vi "Local MS Initialization.vi"(6 "PID Cluster":T2={"L1 to L4 PID Cluster"={"L1 PID Gains"={"Kp"=0.005, "Kd"=0.5, "Ki"=0.0005}, "L2 PID Gains"={"Kp"=0.01, "Kd"=1.0, "Ki"=0.005}, "L3 PID Gains"={"Kp"=0.05, "Kd"=1.0, "Ki"=0.0005}, "L4 PID Gains"={"Kp"=0.1, "Kd"=0.1, "Ki"=0.0005}}, "Stage PID Cluster"={"Stage Z PID"={"Kp"=0.0005, "Kd"=0.001, "Ki"=0.0}, "Stage Y PID"={"Kp"=0.0003, "Kd"=0.01, "Ki"=0.0}, "Stage X PID"={"Kp"=0.0003, "Kd"=0.01, "Ki"=0.0}}, "OCT Z PID Gains"={"Kp"=0.0003, "Kd"=0.0001, "Ki"=0.01}}, 8 "error in":errorcluster, 9 "Offset Home 2 RCM":dbl[](array[numeric])=[0.0, 0.0, 0.0, 0.0], 10 "Prev Posit Cluster":T3={"Prev L1 to L4 Posit"=[0.0, 0.0, 0.0, 0.0], "Prev Stage Posit"=[6.0, 6.0, 6.0], "Prev OCT Z Posit"=0.0}, 11 "FPGA VI Reference In":refnum<k20>) -> (0 "error out":errorcluster, 2 "Last Posit Cluster":T1={"Last L1 to L4 Posit"=[0.0, 0.0, 0.0, 0.0], "Last Stage Posit"=[6.0, 6.0, 6.0], "Last OCT Z Posit"=0.0}, 3 "FPGA VI Reference Out":refnum<k20>)   [LabVIEW 2016]
uses:
  <vilib>/Platform/TimedLoop/XDataNode/timing_clust.ctl
  <vilib>/Platform/TimedLoop/XDataNode/nitl_modes.ctl
  <vilib>/Platform/TimedLoop/XDataNode/wakeup.ctl
  Global Variables.vi
  <vilib>/platform/TimedLoop/XDataNode/XDataNode.xnode
  <vilib>/Platform/TimedLoop/XDataNode/XDNodeRunTimeDep.lvlib
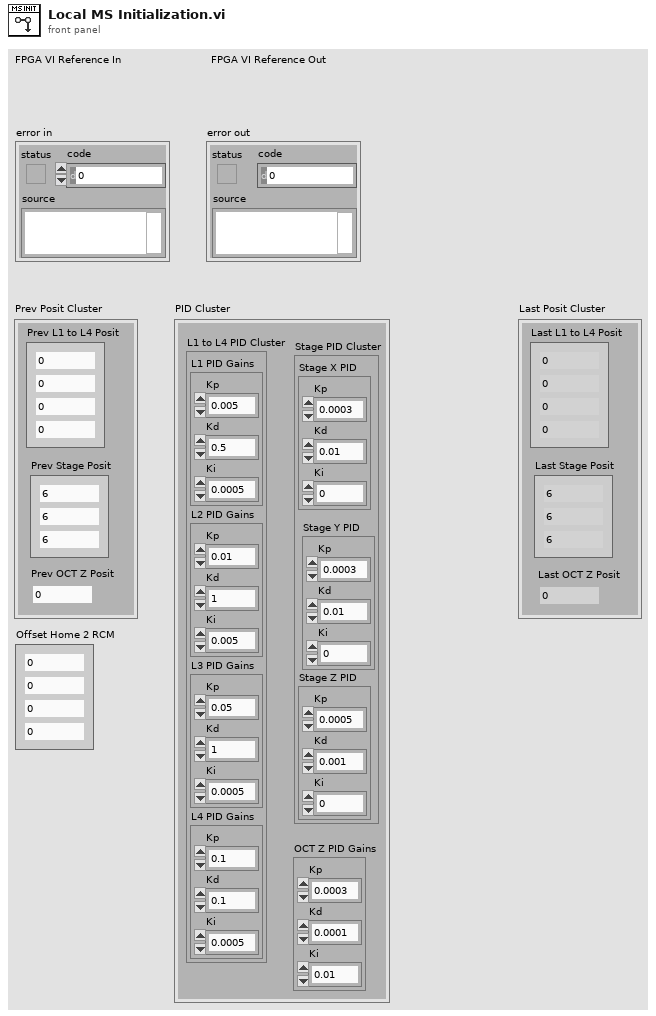
[diagram p1: front panel]
types:
  T1 = cluster{"Last L1 to L4 Posit":dbl[], "Last Stage Posit":dbl[], "Last OCT Z Posit":dbl}
  T2 = cluster{"L1 to L4 PID Cluster":cluster{"L1 PID Gains":cluster{"Kp":dbl, "Kd":dbl, "Ki":dbl}, "L2 PID Gains":cluster{"Kp":dbl, "Kd":dbl, "Ki":dbl}, "L3 PID Gains":cluster{"Kp":dbl, "Kd":dbl, "Ki":dbl}, "L4 PID Gains":cluster{"Kp":dbl, "Kd":dbl, "Ki":dbl}}, "Stage PID Cluster":cluster{"Stage Z PID":cluster{"Kp":dbl, "Kd":dbl, "Ki":dbl}, "Stage Y PID":cluster{"Kp":dbl, "Kd":dbl, "Ki":dbl}, "Stage X PID":cluster{"Kp":dbl, "Kd":dbl, "Ki":dbl}}, "OCT Z PID Gains":cluster{"Kp":dbl, "Kd":dbl, "Ki":dbl}}
  T3 = cluster{"Prev L1 to L4 Posit":dbl[], "Prev Stage Posit":dbl[], "Prev OCT Z Posit":dbl}
  T4 = typedef "XDNodeRunTimeDep.lvlib/timing_clust.ctl" = cluster{"Expected End [f-1]":u64, "Actual End [f-1]":u64, "Finished Late? [f-1]":bool, "Expected End [i-1]":u64, "Actual End [i-1]":u64, "Finished Late? [i-1]":bool, "Expected Start [i]":u64, "Actual Start [i]":u64, "Expected Start [f]":u64, "Actual Start [f]":u64, "Source Name":string, "Structure Name":string, "Period":i64, "Deadline":i64, "Offset":i64, "Start":i64, "Priority":i32, "Timeout":i32, "Mode":T5, "Wakeup Reason":T6, "Error":errorcluster, "Source Type":string, "Secondary Source Type":string, "Global End Time":u64, "Global Start Time":u64, "Frame Duration":u64, "Iteration Duration":u64, "Assigned CPU":i32, "I/O Scan Engine Mode":u32}
  T5 = typedef "XDNodeRunTimeDep.lvlib/nitl_modes.ctl" = enum32{"No Change", "Process missed periods, maintain original phase", "Discard missed periods, maintain original phase", "Process missed periods, ignore original phase", "Discard missed periods, ignore original phase"}
  T6 = typedef "XDNodeRunTimeDep.lvlib/wakeup.ctl" = enum32{"Normal", "Aborted", "Asynchronous wakeup", "Timing source error", "Timed loop error", "Timeout"}
  T7 = cluster{"L1 PID Gains":cluster{"Kp":dbl, "Kd":dbl, "Ki":dbl}, "L2 PID Gains":cluster{"Kp":dbl, "Kd":dbl, "Ki":dbl}, "L3 PID Gains":cluster{"Kp":dbl, "Kd":dbl, "Ki":dbl}, "L4 PID Gains":cluster{"Kp":dbl, "Kd":dbl, "Ki":dbl}}
  T8 = cluster{"Stage Z PID":cluster{"Kp":dbl, "Kd":dbl, "Ki":dbl}, "Stage Y PID":cluster{"Kp":dbl, "Kd":dbl, "Ki":dbl}, "Stage X PID":cluster{"Kp":dbl, "Kd":dbl, "Ki":dbl}}
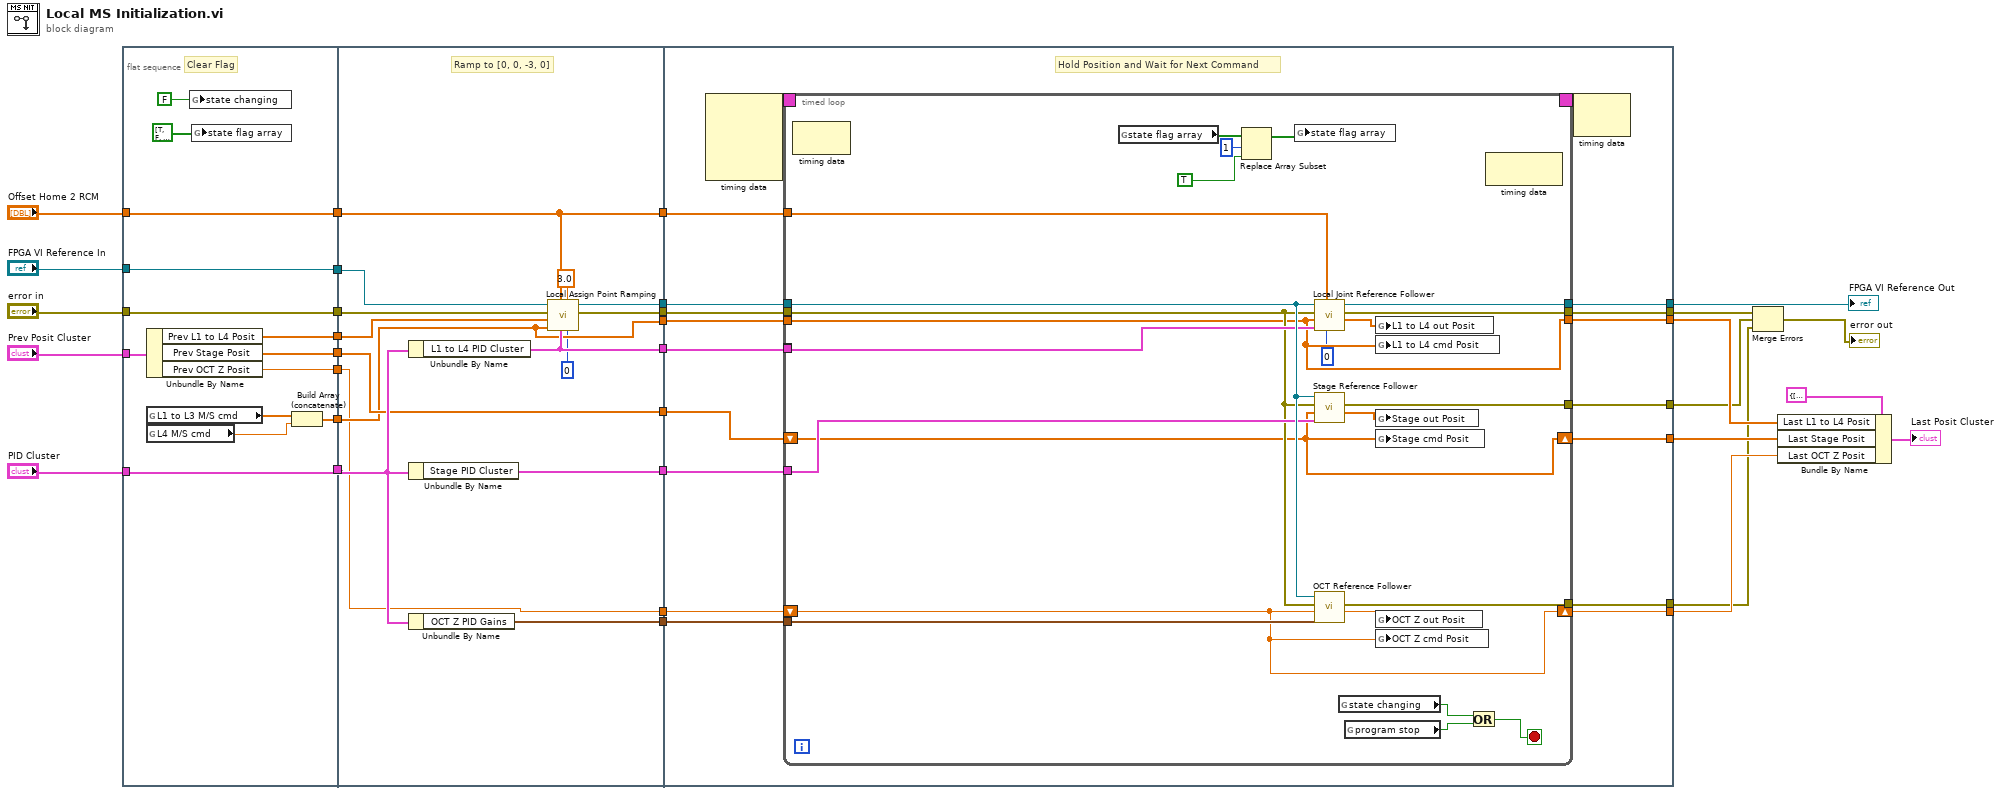
[diagram p0: block diagram]
diagram:
  n1 = flat-sequence {
    tunnel: "Prev Posit Cluster" -> [w43]
    tunnel: [w33] -> w31
    tunnel: [w42] -> w30
    tunnel: [w41] -> w29
    tunnel: "PID Cluster" -> [w41]
    tunnel: "error in" -> [w40]
    tunnel: [w40] -> w26
    tunnel: "Offset Home 2 RCM" -> [w39]
    tunnel: [w39] -> w24
    tunnel: [w38] -> w23
    tunnel: "FPGA VI Reference In" -> [w38]
    tunnel: [w37] -> w4
    tunnel: [w36] -> w2
    tunnel: w31 -> [w48]
    tunnel: w30 -> [w60]
    tunnel: w29 -> [w56]
    tunnel: w26 -> [w59]
    tunnel: w24 -> [w50]
    tunnel: w23 -> [w58]
    tunnel: [w55] -> w21
    tunnel: [w54] -> w20
    tunnel: [w53] -> w19
    tunnel: [w52] -> w18
    tunnel: [w51] -> w17
    tunnel: [w48] -> w16
    tunnel: [w50] -> w15
    tunnel: w4 -> [w49]
    tunnel: [w49] -> w3
    tunnel: w2 -> [w46]
    tunnel: [w46] -> w1
    tunnel: w21 -> [w76]
    tunnel: w20 -> [w75]
    tunnel: w19 -> [w74]
    tunnel: w18 -> [w73]
    tunnel: w17 -> [w72]
    tunnel: w16 -> [w71]
    tunnel: w15 -> [w70]
    tunnel: [w69] -> w14
    tunnel: [w68] -> w8
    tunnel: [w67] -> w11
    tunnel: [w66] -> w10
    tunnel: [w65] -> w9
    tunnel: [w64] -> w6
    tunnel: [w63] -> w5
    tunnel: w3 -> [w62]
    tunnel: w1 -> [w61]
    frame #0 {
      # "Clear Flag"
      n2 = Unbundle By Name(w43) -> ("Prev L1 to L4 Posit"=w42:dbl[], "Prev Stage Posit"=w37:dbl[], "Prev OCT Z Posit"=w36:dbl)
      n3 = global read "Global Variables.vi" "L1 to L3 M/S cmd"() -> (w35:dbl[])
      n4 = global read "Global Variables.vi" "L4 M/S cmd"() -> (w34:dbl)
      n5 = global write "Global Variables.vi" "state changing"(FALSE ("state changing")) -> ()
      n6 = global write "Global Variables.vi" "state flag array"(bool[] [TRUE, FALSE, FALSE, FALSE, FALSE, FALSE, FALSE, FALSE, FALSE] ("state flag array")) -> ()
      n7 = Build Array (concatenate)(w35, w34) -> (w33:dbl[])
    }
    frame #1 {
      # "Ramp to [0, 0, -3, 0]"
      n8 = Unbundle By Name(w56) -> ("L1 to L4 PID Cluster"=w53:T7)
      n9 = Unbundle By Name(w56) -> ("Stage PID Cluster"=w52:T8)
      n10 = Unbundle By Name(w56) -> ("OCT Z PID Gains"=w51:cluster{"Kp":dbl, "Kd":dbl, "Ki":dbl})
      n11 = call "Local Assign Point Ramping.vi"("Vac Digital Cmd"=i8 0, "Ramp Time [sec]"=3.0, "L1 to L4 PID Cluster"=w53, "Offset Home2RCM"=w50, "Destination Posit Array [mm]"=w48, "Previous Posit Array"=w60, "error in"=w59, "FPGA VI Reference In"=w58) -> ("error out"=w54:errorcluster, "FPGA VI Reference Out"=w55:refnum<k20>)  [unwired: 1 in, 1 out]
    }
    frame #2 {
      # "Hold Position and Wait for Next Command"
      n12 = node-c288() -> (w78:T4)  [unwired: 4 in]
      n13 = timed-loop {
        timing: w78 -> [_]
        timing-out: [_] -> w77
        tunnel: w76 -> [w95]
        tunnel: w75 -> [w91]
        tunnel: [w94] -> _
        tunnel: w74 -> [w94]
        tunnel: w73 -> [w93]
        tunnel: w72 -> [w92]
        tunnel: w71 -> [w82]
        tunnel: w70 -> [w90]
        tunnel: [w89] -> w69
        tunnel: [w88] -> w68
        tunnel: [w82] -> w67
        tunnel: [w84] -> w64
        tunnel: [w83] -> w63
        shift-right: [w81] -> w66
        shift-left: w62 -> [w81]
        shift-right: [w80] -> w65
        shift-left: w61 -> [w80]
        stop <- w102 stop-if-true
        n14 = node-c288() -> ()  [unwired: 1 in, 1 out]
        n15 = global read "Global Variables.vi" "state flag array"() -> (w99:bool[])
        n16 = Replace Array Subset(array=w99, new element=TRUE ("new element/subarray"), index=1) -> (w98:bool[])
        n17 = global write "Global Variables.vi" "state flag array"(w98) -> ()
        n18 = call "Local Joint Reference Follower.vi"("Digital Cmd [0-78]"=i8 0 ("Vac Digital Cmd"), "Offset Home2RCM [deg/mm]"=w90, "PID Ctrl Cluster"=w94, "Ref Array [deg/mm]"=w82, "error in"=w91, "FPGA VI Reference In"=w95) -> ("Output Posit Array [deg/mm]"=w87:dbl[], "error out"=w88:errorcluster, "FPGA VI Reference Out"=w89:refnum<k20>)  [unwired: 3 in]
        n19 = call "Stage Reference Follower.vi"("Stage PID Cluster"=w93, "Stage cmd Posit [mm]"=w81, "error in"=w91, "FPGA VI Reference In"=w95) -> ("Stage out Posit [mm]"=w86:dbl[], "error out"=w84:errorcluster)  [unwired: 5 in, 1 out]
        n20 = call "OCT Reference Follower.vi"("OCT Z PID Gains"=w92, "OCT  Z cmd Posit [mm]"=w80, "error in"=w91, "FPGA VI Reference In"=w95) -> ("OCT  Z out Posit [mm]"=w85:dbl, "error out"=w83:errorcluster)  [unwired: 5 in, 1 out]
        n21 = global read "Global Variables.vi" "state changing"() -> (w101:bool)
        n22 = global read "Global Variables.vi" "program stop"() -> (w100:bool)
        n23 = global write "Global Variables.vi" "L1 to L4 out Posit"(w87) -> ()
        n24 = global write "Global Variables.vi" "L1 to L4 cmd Posit"(w82) -> ()
        n25 = global write "Global Variables.vi" "Stage out Posit"(w86) -> ()
        n26 = global write "Global Variables.vi" "Stage cmd Posit"(w81) -> ()
        n27 = global write "Global Variables.vi" "OCT Z out Posit"(w85) -> ()
        n28 = global write "Global Variables.vi" "OCT Z cmd Posit"(w80) -> ()
        n29 = Or(x=w101, y=w100) -> (x .or. y?=w102:bool)
        n30 = node-c288() -> ()  [unwired: 1 in, 1 out]
      }
      n31 = node-c288(w77) -> ()  [unwired: 1 out]
    }
  }
  n32 = Merge Errors(w8, w6, w5) -> (→"error out":errorcluster)
  n33 = Bundle By Name(cluster=T1 {"Last L1 to L4 Posit"=[0.0, 0.0, 0.0, 0.0], "Last Stage Posit"=[6.0, 6.0, 6.0], "Last OCT Z Posit"=0.0} ("Last Posit Cluster 2"), "Last L1 to L4 Posit"=w11, "Last Stage Posit"=w10, "Last OCT Z Posit"=w9) -> (→"Last Posit Cluster":T1)
  "FPGA VI Reference Out" <- w14
